vi "Save Orientation History.vi"() -> (2 "File Name refnum":refnum<file>, 3 "File Name path":path)   [LabVIEW 2016]
uses:
  navxmxp/roborio/labviewae/_TypeDefs/FRIC_navX_DeviceNumbersTypeDef.ctl
  <vilib>/Utility/file.llb/Write Delimited Spreadsheet (DBL).vi
panel:
  out "iterations":i32
  out "size(s)":i32[](array[numeric])
  in  "Device Number":T1
  out "error out":errorcluster
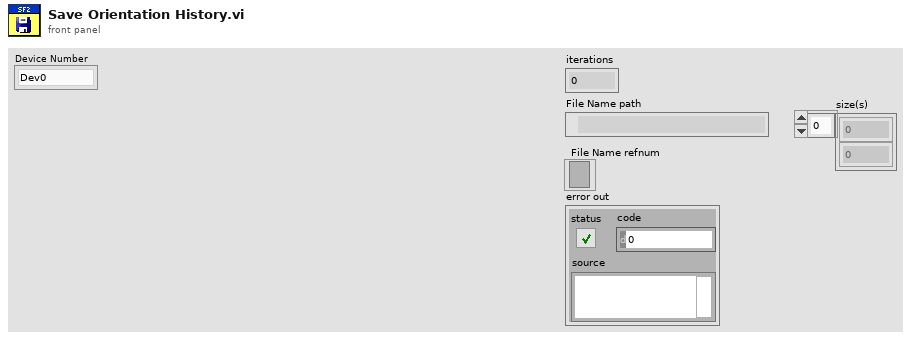
[diagram p1: front panel]
types:
  T1 = typedef "FRIC_navX_DeviceNumbersTypeDef.ctl" = enum16{"Dev0", "Dev1", "Dev2", "Dev3"}
  T2 = enum16{"open", "replace", "create", "open or create", "replace or create", "replace or create with confirmation"}
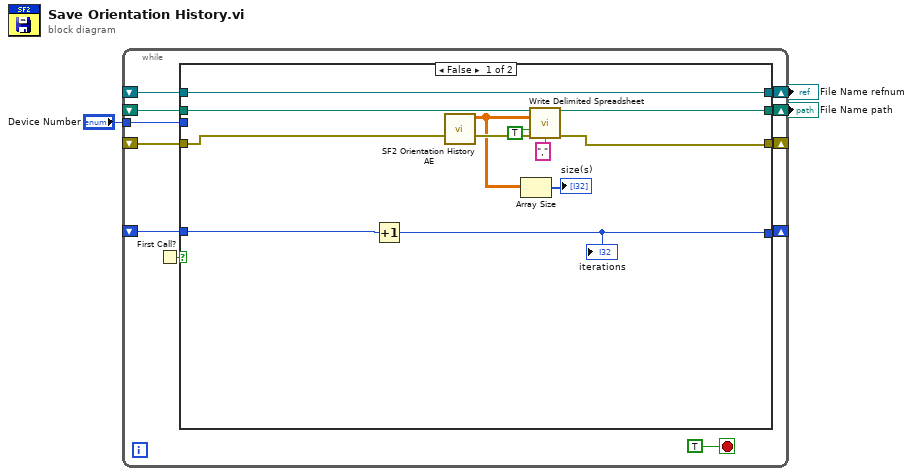
[diagram p0: block diagram]
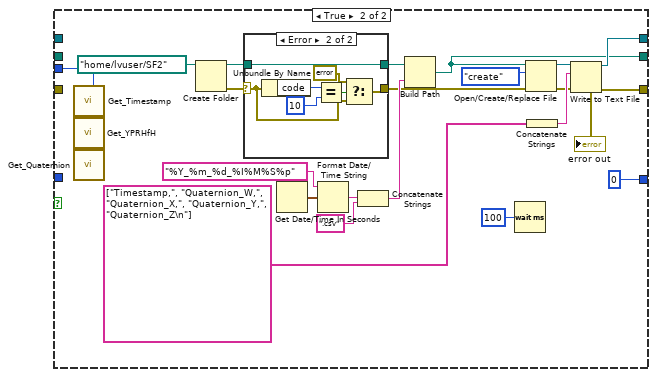
[diagram p2: hidden frame]
diagram:
  n1 = while {
    shift-right: [w14] -> w3
    shift-left: _ -> [w10]
    shift-right: [w13] -> _
    shift-left: _ -> [w9]
    shift-right: [w8] -> w2
    shift-left: _ -> [w7]
    tunnel: "Device Number" -> [w6]
    shift-right: [w5] -> _
    shift-left: _ -> [w4]
    stop <- TRUE stop-if-true
    n2 = First Call?() -> (First Call?: T/F=w11:bool)
    n3 = case shown="False" w11 {
      tunnel: [w23 w35] -> w14
      tunnel: [w22 w34] -> w13
      tunnel: w10 -> [w23 _]
      tunnel: w9 -> [w21 _]
      tunnel: [w24 w29] -> w8
      tunnel: w7 -> [w25 _]
      tunnel: w6 -> [_ w28]
      tunnel: [w15 0] -> w5
      tunnel: w4 -> [w16 _]
      frame False {
        n4 = Increment(x=w16) -> (x+1=w15:i32)
        "iterations" <- w15
        n5 = call "SF2 Orientation History AE.vi"() -> ("SF2 Buffer (out)"=w18:dbl[][])  [unwired: 11 in]
        n6 = Array Size(array=w18) -> (size(s)=→"size(s)":i32[])
        n7 = call-poly <vilib>:"Write Delimited Spreadsheet.vi"("file path (dialog if empty)"=w25, "2D data"=w18, "append to file? (new file:F)"=TRUE, "error in (no error)"=w21, "delimiter (\\t)"="," ("delimiter (\\t)")) -> ("new file path (Not A Path if cancelled)"=w24:path, "error out"=w22:errorcluster)  [unwired: 9 in]
      }
      frame True {
        n8 = call "Get_Timestamp.vi"("Device Number"=w28) -> ()  [unwired: 10 in, 1 out]
        n9 = call "Get_YPRHfH.vi"("Device Number"=w28) -> ()  [unwired: 10 in, 1 out]
        n10 = call "Get_Quaternion.vi"("Device Number"=w28) -> ()  [unwired: 10 in, 1 out]
        n11 = Create Folder(path (use dialog)=path "/home/lvuser/SF2") -> (created path=w30:path, error out=w33:errorcluster)  [unwired: 2 in, 1 out]
        n12 = case shown="Error" w33 {
          selector: w33 -> [w47 w51]
          tunnel: w30 -> [w48 w55]
          tunnel: [w48 w55] -> w32
          tunnel: [w47 w50] -> w31
          frame No Error {
          }
          frame Error {
            n13 = Unbundle By Name(w51) -> ("code"=w54:i32)
            n14 = Equal?(x=w54, y=10) -> (x = y?=w49:bool)
            n15 = Select(t=errorcluster {"status"=FALSE, "code"=0, "source"=""} ("error IO"), s=w49, f=w51) -> (s? t:f=w50:errorcluster)
          }
        }
        n16 = Get Date/Time In Seconds() -> (seconds since 1Jan1904=w42:timestamp)
        n17 = Format Date/Time String(time format string (%c)="%Y_%m_%d_%I%M%S%p", seconds (now)=w42) -> (date/time string=w43:string)  [unwired: 1 in]
        n18 = Concatenate Strings(w43, ".csv" ("string")) -> (w40:string)
        n19 = Build Path(base path=w32, name or relative path=w40) -> (appended path=w29:path)
        n20 = Wait (ms)(milliseconds to wait=u32 100) -> ()  [unwired: 1 out]
        n21 = Open/Create/Replace File(file path (use dialog)=w29, error in=w31, operation (0:open)=T2."create") -> (refnum out=w39:refnum<file>, error out=w36:errorcluster)  [unwired: 3 in, 1 out]
        n22 = Concatenate Strings(string[] ["Timestamp,", "Quaternion_W,", "Quaternion_X,", "Quaternion_Y,", "Quaternion_Z\n"]) -> (w37:string)
        n23 = Write to Text File(file (use dialog)=w39, text=w37, error in=w36) -> (refnum out=w35:refnum<file>, error out=w34:errorcluster)  [unwired: 1 in, 1 out]
        "error out" <- w34
      }
    }
  }
  "File Name refnum" <- w3
  "File Name path" <- w2
